vi "test queues and notifiers.vi"() -> ()   [LabVIEW 2019]
panel:
  in  "stop":bool
  out "latest notification":string
  in  "notification":string
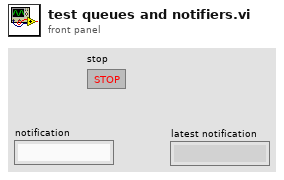
[diagram p1: front panel]
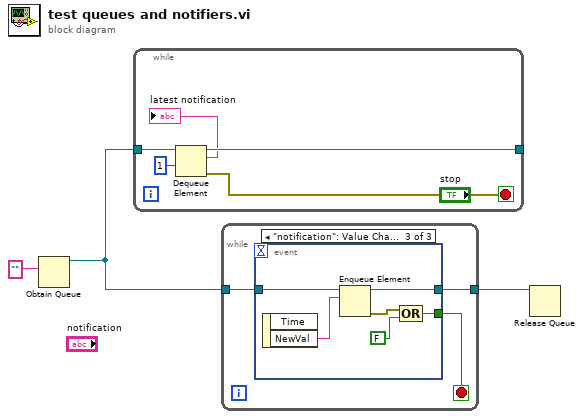
[diagram p0: block diagram]
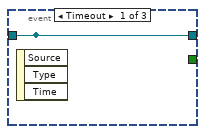
[diagram p2: hidden frame]
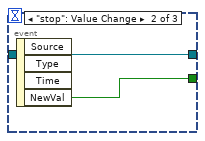
[diagram p3: hidden frame]
diagram:
  n1 = Obtain Queue(element data type="") -> (queue out=w2:refnum<queue>)  [unwired: 4 in, 2 out]
  n2 = while {
    tunnel: w2 -> [w8]
    tunnel: [w7] -> _
    stop <- w5 stop-if-true
    n3 = Dequeue Element(queue=w8, timeout in ms (-1)=1) -> (queue out=w7:refnum<queue>, element=→"latest notification":string, error out=w5:errorcluster)  [unwired: 1 in, 1 out]
  }
  n4 = while {
    tunnel: w2 -> [w11]
    tunnel: [w9] -> w1
    stop <- w10 stop-if-true
    n5 = event shown="[2] \"notification\": Value Change" {
      selector: _ -> [_ _ _]
      dyn-events: _ -> [_ _ _]
      timeout: _ -> [_ _ _]
      tunnel: w11 -> [w12 w13 w20]
      tunnel: [w12 _ _] -> _
      tunnel: [_ w14 w16] -> w10
      tunnel: [w12 w13 w15] -> w9
      event Timeout {
        n6 = event-data() -> ()  [unwired: 1 in, 3 out]
      }
      event "stop": Value Change {
        n7 = event-data() -> ("NewVal"=w14:bool)  [unwired: 1 in, 3 out]
      }
      event "notification": Value Change {
        n8 = event-data() -> ("NewVal"=w19:string)  [unwired: 1 in, 1 out]
        n9 = Enqueue Element(queue=w20, element=w19) -> (queue out=w15:refnum<queue>, error out=w17:errorcluster)  [unwired: 2 in, 1 out]
        n10 = Compound Arithmetic op=OR(w17, FALSE) -> (w16:bool)
      }
    }
  }
  n11 = Release Queue(queue=w1) -> ()  [unwired: 2 in, 3 out]
